vi "samples.vi"(3 "elemszam":u8) -> ()   [LabVIEW 2014]
uses:
  <vilib>/Analysis/NI_AALBase.lvlib
panel:
  out "Sinusoidal Pattern":dbl[](array[numeric])
  out "Waveform Chart":dbl[](graph)
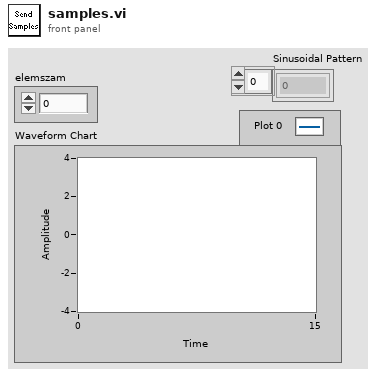
[diagram p1: front panel]
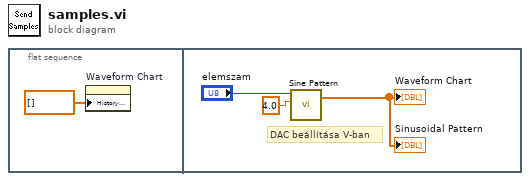
[diagram p0: block diagram]
diagram:
  n1 = flat-sequence {
    frame #0 {
      n2 = property on="Waveform Chart" class="WFChart (strict)"("History Data"=dbl[] []) -> ()  [unwired: 2 in, 2 out]
    }
    frame #1 {
      # "DAC beállítása V-ban"
      n3 = call <vilib>:"Sine Pattern.vi"("amplitude"=4.0, "samples"="elemszam") -> ("Sinusoidal Pattern"=→"Waveform Chart" →"Sinusoidal Pattern":dbl[])  [unwired: 2 in, 1 out]
    }
  }
